vi "Fail If.vi"(7 "Description":string, 8 "error in (no error)":errorcluster, 9 "Message":string, 10 "Fail?":bool, 11 "LUnit Test Case In":refnum<class "LUnit Inheriting Test Case.lvclass">) -> (0 "error out":errorcluster, 3 "LUnit Test Case Out":refnum<class "LUnit Inheriting Test Case.lvclass">)   [LabVIEW 2020]
doc: "Generates a fail result for the calling test method if the conditional input is true. A description and message may be provided."
uses:
  LUnit Inheriting Test Case.lvclass
  Core/Result/Type.ctl
  Core/Result/Result.lvlib
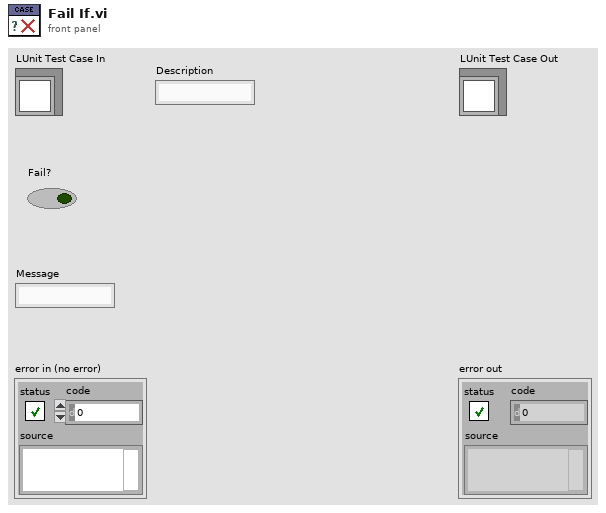
[diagram p1: front panel]
types:
  T1 = typedef "Result.lvlib/Type.ctl" = enum16{"Test Case", "Test Suite", "Test Run", "Pass", "Fail", "Skip", "Pass if", "Fail if", "Pass if Error", "Fail if Error", "Pass if Equal", "Fail if Equal"}
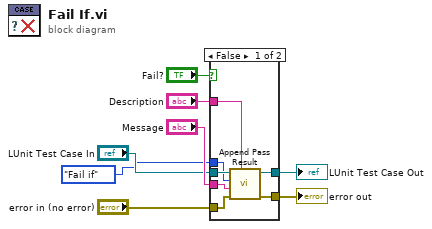
[diagram p0: block diagram]
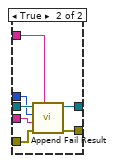
[diagram p2: hidden frame]
diagram:
  n1 = case shown="False" "Fail?" {
    tunnel: [w15 w21] -> w8
    tunnel: [w11 w20] -> w4
    tunnel: "Description" -> [w13 w18]
    tunnel: "Message" -> [w12 w19]
    tunnel: "LUnit Test Case In" -> [w14 w22]
    tunnel: "error in (no error)" -> [w10 w17]
    tunnel: Type."Fail if" ("Result Type") -> [w9 w16]
    frame False {
      n2 = call "Append Pass Result.vi"("Description"=w13, "error in (no error)"=w10, "Message"=w12, "Result Type"=w9, "LUnit Test Case In"=w14) -> ("error out"=w11:errorcluster, "LUnit Test Case Out"=w15:refnum<class "LUnit Inheriting Test Case.lvclass">)  [unwired: 5 in]
    }
    frame True {
      n3 = call "Append Fail Result.vi"("Description"=w18, "error in (no error)"=w17, "Message"=w19, "Result Type"=w16, "LUnit Test Case In"=w22) -> ("error out"=w20:errorcluster, "LUnit Test Case Out"=w21:refnum<class "LUnit Inheriting Test Case.lvclass">)  [unwired: 5 in]
    }
  }
  "error out" <- w4
  "LUnit Test Case Out" <- w8
